vi "Search DS402 device.vi"(8 "error in (no error)":errorcluster, 11 "Slave Reference In":refnum<k21>) -> (0 "error out":errorcluster, 2 "Found":bool, 3 "Slave Reference Out":refnum<k21>)   [LabVIEW 2016, in "Scan Engine Custom Device.lvlib"]
uses:
  Scan Engine Custom Device.lvlib
  <resource>/objmgr/IndComECAT.rc
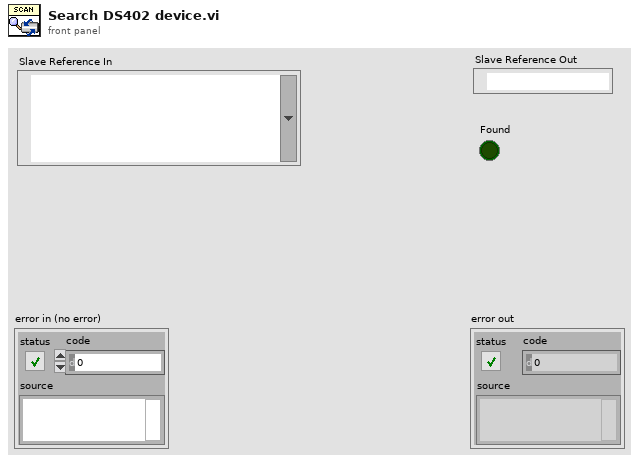
[diagram p1: front panel]
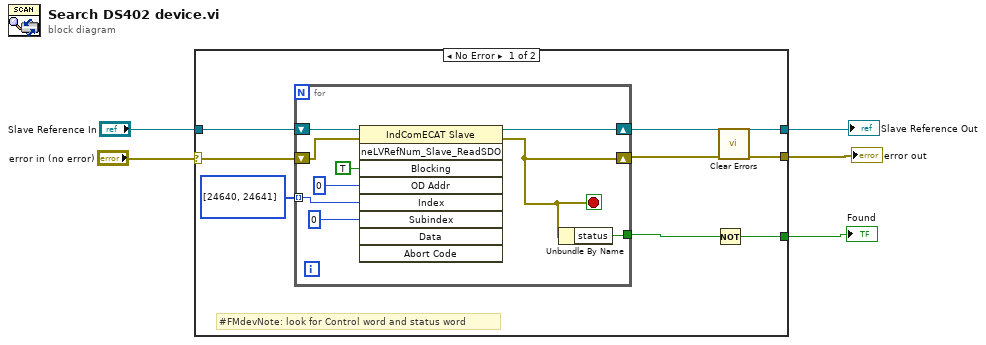
[diagram p0: block diagram]
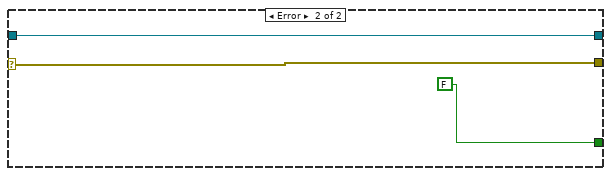
[diagram p2: hidden frame]
diagram:
  n1 = case shown="No Error" "error in (no error)" {
    selector: "error in (no error)" -> [w12 w25]
    tunnel: "Slave Reference In" -> [w13 w24]
    tunnel: [w6 w25] -> w3
    tunnel: [w8 w24] -> w2
    tunnel: [w9 FALSE] -> w1
    frame No Error {
      # "#FMdevNote: look for Control word and status word"
      n2 = for {
        shift-right: [w19] -> w8
        shift-left: w13 -> [w21]
        tunnel: u16[] [24640, 24641] ("OD Addr") -> [w14] mode=indexing
        shift-right: [w18] -> w7
        shift-left: w12 -> [w22]
        tunnel: [w17] -> w10
        stop <- w18 stop-if-true
        n3 = invoke class="IndComECAT Slave" method="neLVRefNum_Slave_ReadSDO"(reference=w21, error in=w22, "Blocking"=TRUE, "OD Addr"=u16 0, "Index"=w14, "Subindex"=u16 0 ("Index")) -> (reference out=w19:refnum<k21>, error out=w18:errorcluster)  [unwired: 3 in, 7 out]
        n4 = Unbundle By Name(w18) -> ("status"=w17:bool)
      }
      n5 = Not(x=w10) -> (.not. x?=w9:bool)
      n6 = call <vilib>:"Clear Errors.vi"("error in (no error)"=w7) -> ("error out"=w6:errorcluster)  [unwired: 5 in, 1 out]
    }
    frame Error {
    }
  }
  "error out" <- w3
  "Found" <- w1
  "Slave Reference Out" <- w2
